vi "Error Test Label Count.vi"(6 "error text in":string, 8 "error in":errorcluster, 10 "number of labels":i32) -> (0 "error out":errorcluster)   [LabVIEW 2024]
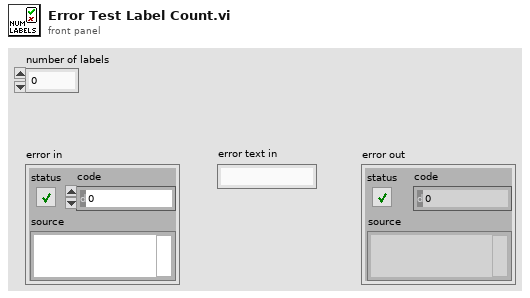
[diagram p1: front panel]
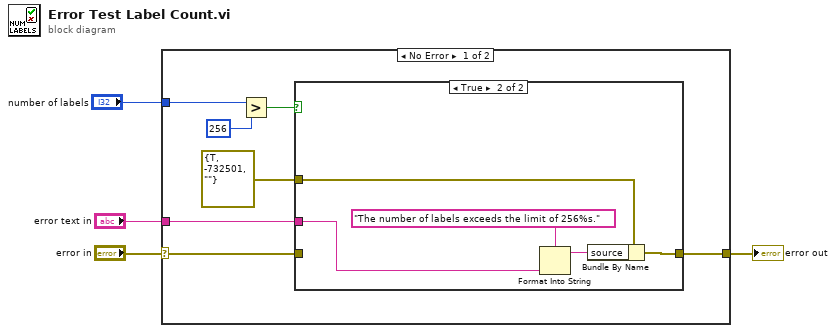
[diagram p0: block diagram]
diagram:
  n1 = case shown="No Error" "error in" {
    selector: "error in" -> [w9 w18]
    tunnel: [w11 w18] -> w3
    tunnel: "error text in" -> [w6 _]
    tunnel: "number of labels" -> [w5 _]
    frame No Error {
      n2 = Greater?(x=w5, y=256) -> (0:w7:bool)
      n3 = case shown="True" w7 {
        tunnel: errorcluster {"status"=TRUE, "code"=-732501, "source"=""} ("error constant") -> [_ w16]
        tunnel: [w12 w17] -> w11
        tunnel: w9 -> [w12 _]
        tunnel: w6 -> [_ w13]
        frame False {
        }
        frame True {
          n4 = Format Into String(format string="The number of labels exceeds the limit of 256%s." ("source"), w13) -> (resulting string=w15:string)  [unwired: 2 in, 1 out]
          n5 = Bundle By Name(cluster=w16, "source"=w15) -> (w17:errorcluster)
        }
      }
    }
    frame Error {
    }
  }
  "error out" <- w3
